vi "Centroid.vi"(3 "Points":sgl[][](array[numeric])) -> (0 "Centroid":sgl[](array[numeric]), 1 "Offset vectors":sgl[][](array[numeric]))   [LabVIEW 2013]
panel:
  # "Given some points, return the centroid (mean poisition) and the offsets of the points from that centroid."
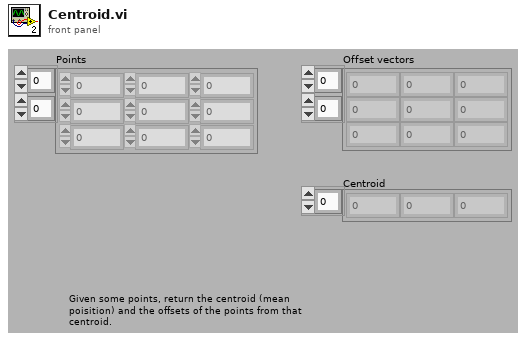
[diagram p1: front panel]
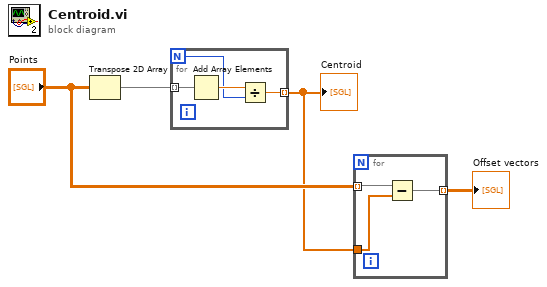
[diagram p0: block diagram]
diagram:
  n1 = Transpose 2D Array(2D array="Points") -> (transposed array=w4:sgl[][])
  n2 = for {
    N -> [w6]
    tunnel: w4 -> [w8] mode=indexing
    tunnel: [w5] -> w2 mode=indexing
    n3 = Add Array Elements(numeric array=w8) -> (sum=w7:sgl)
    n4 = Divide(x=w7, y=w6) -> (x/y=w5:sgl)
  }
  "Centroid" <- w2
  n5 = for {
    tunnel: "Points" -> [w11] mode=indexing
    tunnel: w2 -> [w10]
    tunnel: [w9] -> w1 mode=indexing
    n6 = Subtract(x=w11, y=w10) -> (x-y=w9:sgl[])
  }
  "Offset vectors" <- w1
